vi "GetClassInfo.vi"(0 "ClassWriterNative":refnum<class "ClassWriterNative.lvclass">, 5 "error in (no error)":errorcluster) -> (14 "ClassWriterNative":refnum<class "ClassWriterNative.lvclass">, 15 "LvClassPath":path, 16 "ClassRefnumOut":refnum<vi>, 17 "ProjectRefnum":refnum<vi>, 18 "LvClassFolderPath":path, 19 "error out":errorcluster)   [LabVIEW 2020, in "ClassWriterNative.lvclass"]
uses:
  ClassWriterNative.lvclass
  ClassWriterNative.lvclass/ClassWriterNative.ctl
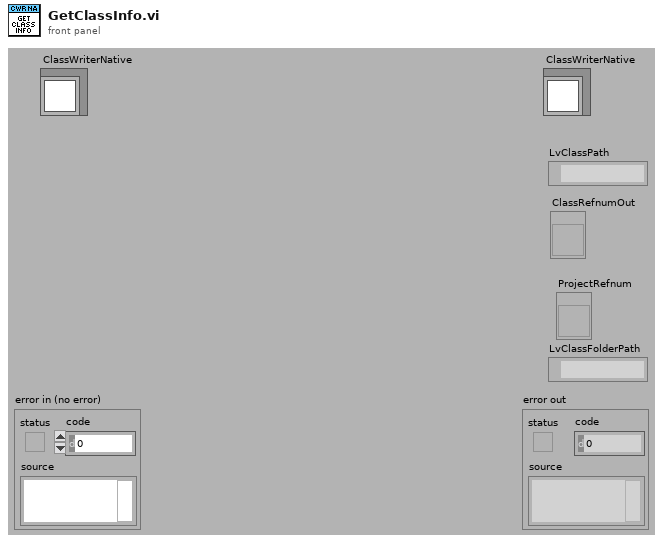
[diagram p1: front panel]
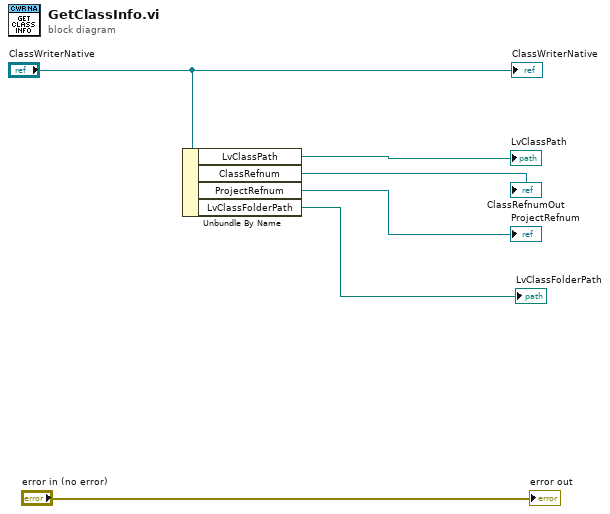
[diagram p0: block diagram]
diagram:
  n1 = Unbundle By Name("ClassWriterNative") -> ("LvClassPath"=→"LvClassPath":path, "ClassRefnum"=→"ClassRefnumOut":refnum<vi>, "ProjectRefnum"=→"ProjectRefnum":refnum<vi>, "LvClassFolderPath"=→"LvClassFolderPath":path)
  "ClassWriterNative" <- "ClassWriterNative"
  "error out" <- "error in (no error)"
